vi "Run Command.vi"(6 "Gantry In":refnum<class "Gantry Class.lvclass">, 7 "Console Log In":refnum<class "Console Log.lvclass">, 8 "error in (no error)":errorcluster, 10 "Command":string, 11 "gScript Interpreter In":refnum<class "gScript Interpreter.lvclass">) -> (0 "error out":errorcluster, 3 "gScript Interpreter Out":refnum<class "gScript Interpreter.lvclass">, 4 "Gantry Out":refnum<class "Gantry Class.lvclass">, 5 "Console Log Out":refnum<class "Console Log.lvclass">)   [LabVIEW 2017, in "gScript Interpreter.lvclass"]
uses:
  gScript Interpreter.lvclass
  Shared Components/Gantry Class/Gantry Class.lvclass
  Application Utilities/Console Log/Console Log.lvclass
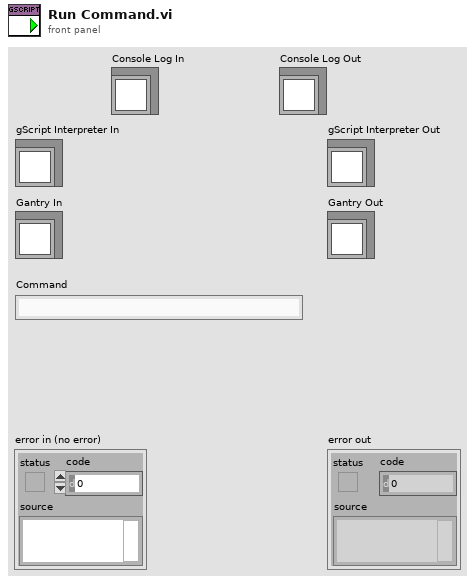
[diagram p1: front panel]
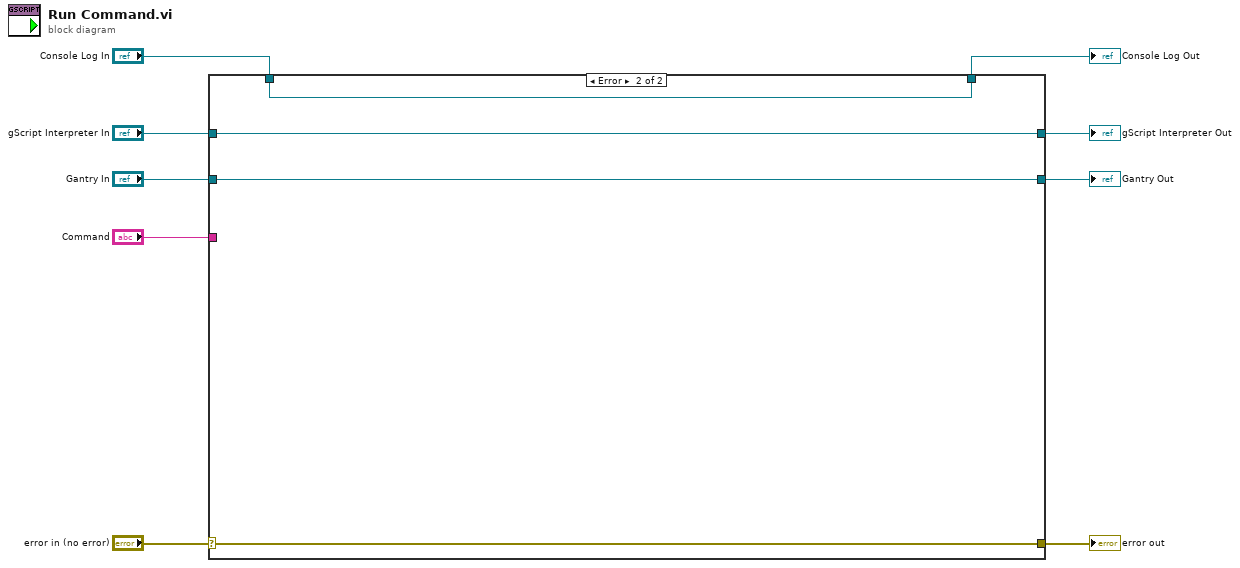
[diagram p0: block diagram]
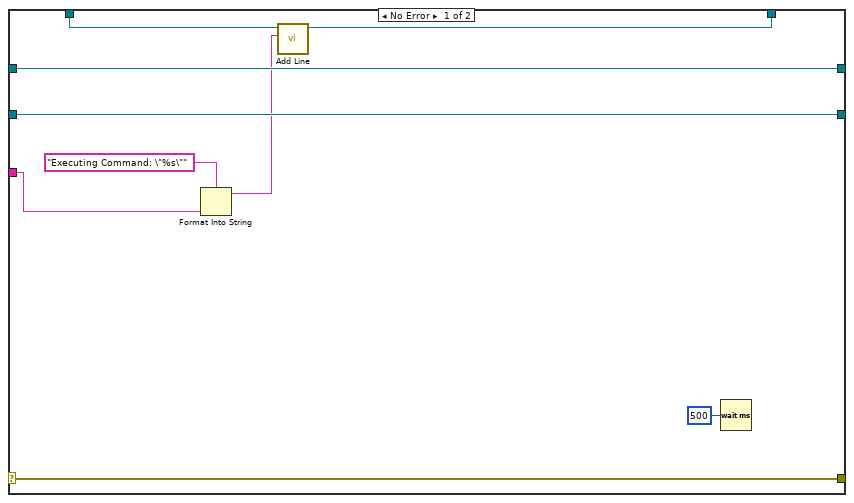
[diagram p2: hidden frame]
diagram:
  n1 = case shown="Error" "error in (no error)" {
    selector: "error in (no error)" -> [w17 w22]
    tunnel: [w17 w22] -> w8
    tunnel: [w18 w21] -> w6
    tunnel: "gScript Interpreter In" -> [w18 w21]
    tunnel: "Console Log In" -> [w15 w20]
    tunnel: [w14 w20] -> w4
    tunnel: "Command" -> [w10 _]
    tunnel: "Gantry In" -> [w16 w19]
    tunnel: [w16 w19] -> w1
    frame No Error {
      n2 = Format Into String(format string="Executing Command: \"%s\"", w10) -> (resulting string=w12:string)  [unwired: 2 in, 1 out]
      n3 = call "Add Line.vi"("String"=w12, "Console Log in"=w15) -> ("Console Log out"=w14:refnum<class "Console Log.lvclass">)  [unwired: 8 in, 1 out]
      n4 = Wait (ms)(milliseconds to wait=u32 500) -> ()  [unwired: 1 out]
    }
    frame Error {
    }
  }
  "error out" <- w8
  "gScript Interpreter Out" <- w6
  "Console Log Out" <- w4
  "Gantry Out" <- w1
